vi "CleanUp.vi"(8 "error in (no error)":errorcluster, 11 "Prueba01 in":refnum<class "Prueba01.lvclass">) -> (0 "error out":errorcluster, 3 "Prueba01 out":refnum<class "Prueba01.lvclass">)   [LabVIEW 2019, in "Prueba01.lvclass"]
uses:
  Prueba01.lvclass
  C:/Users/ivan_/Documents/procal/Pruebas/Prueba/Prueba.lvclass
  Prueba/Prueba.lvclass/Prueba.ctl
  Prueba01.lvclass/Prueba01.ctl
  Base de Datos/SQLiteConnector/SQLiteConnection.lvclass
  Base de Datos/Base de Datos.lvclass
  Prueba/Prueba.lvclass
panel:
  # "estos daros\nse escribirán en la base de datos"
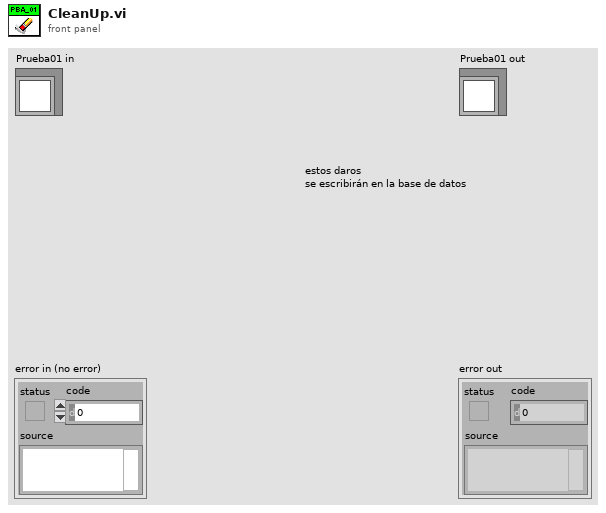
[diagram p1: front panel]
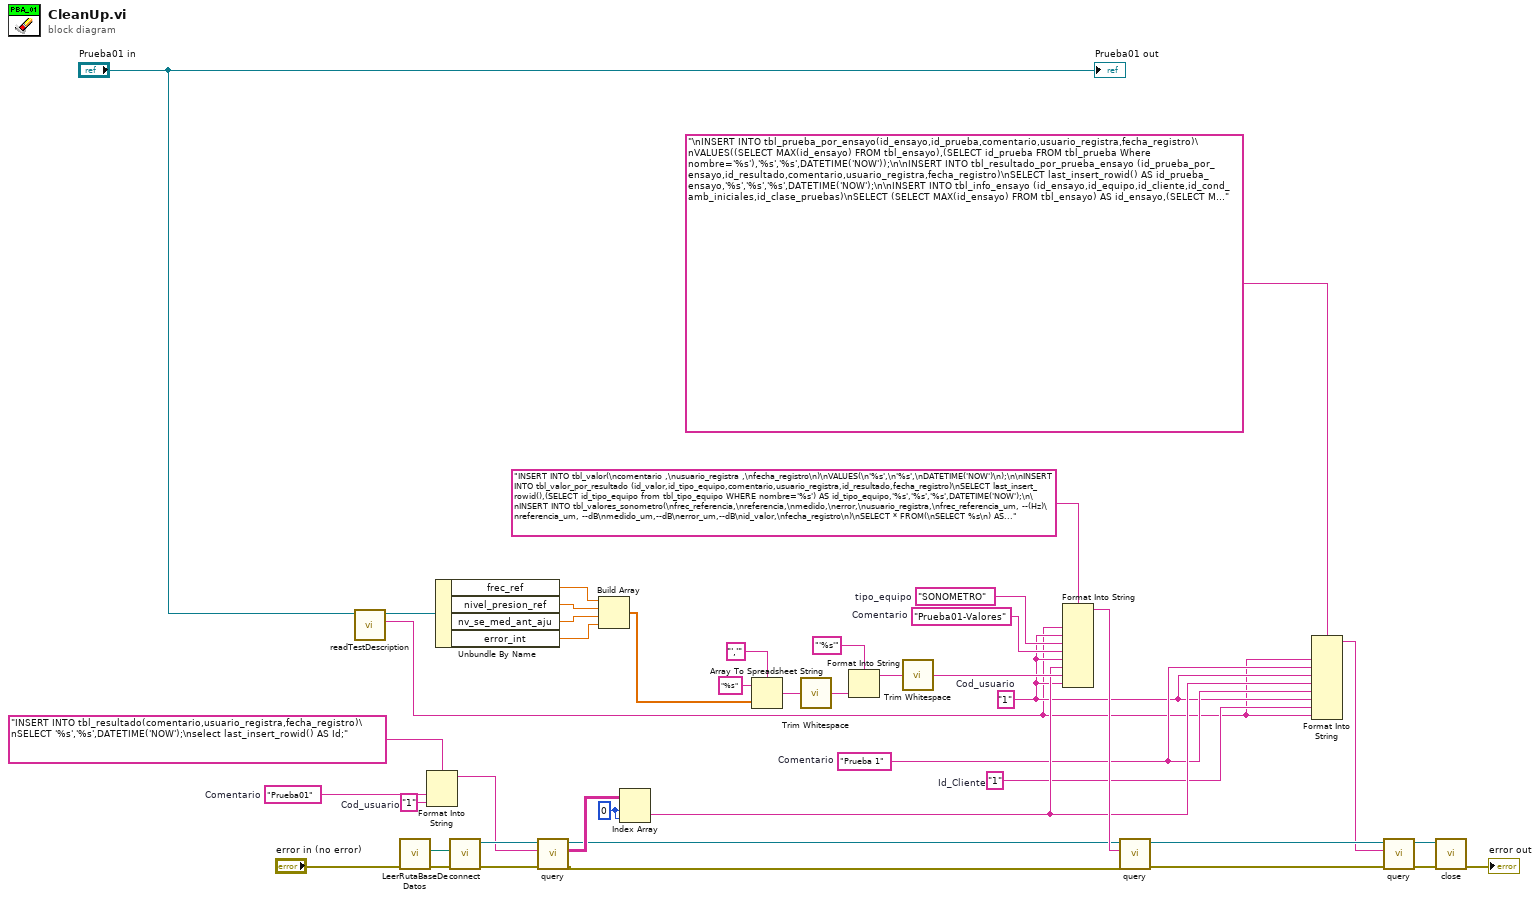
[diagram p0: block diagram]
diagram:
  w18 = "1"  # Id_Cliente
  w19 = "Prueba 1"  # Comentario
  w28 = "SONOMETRO"  # tipo_equipo
  w27 = "Prueba01-Valores"  # Comentario
  w34 = 0 ("index (row)")
  w36 = "1"  # Cod_usuario
  w37 = "Prueba01"  # Comentario
  w15 = "1"  # Cod_usuario
  n1 = call "readTestDescription.vi"("Prueba in"="Prueba01 in") -> ("Test Description"=w2:string, "Prueba out"=w1:refnum<class "Prueba01.lvclass">)  [unwired: 8 in, 1 out]
  n2 = call "LeerRutaBaseDeDatos.vi"("error in (no error)"="error in (no error)") -> ("error out"=w42:errorcluster, "Database Path"=w41:path)  [unwired: 9 in]
  n3 = Format Into String(format string="INSERT INTO tbl_resultado(comentario,usuario_registra,fecha_registro)\nSELECT '%s','%s',DATETIME('NOW');\nselect last_insert_rowid() AS Id;" ("SQL Statement"), w37, w36) -> (resulting string=w35:string)  [unwired: 2 in, 1 out]
  n4 = Unbundle By Name(w1) -> ("frec_ref"=w6:dbl, "nivel_presion_ref"=w7:dbl, "nv_se_med_ant_aju"=w8:dbl, "error_int"=w9:dbl)
  n5 = call "connect.vi"("error in (no error)"=w42, "Database Path"=w41) -> ("error out"=w33:errorcluster, "object out"=w39:refnum<class "SQLiteConnection.lvclass">)  [unwired: 8 in]
  n6 = call "query.vi"("error in (no error)"=w33, "SQL Statement"=w35, "object in"=w39) -> ("error out"=w30:errorcluster, "result"=w32:string[][], "object out"=w31:refnum<class "SQLiteConnection.lvclass">)  [unwired: 5 in, 1 out]
  n7 = Build Array(w6, w7, w8, w9) -> (w5:dbl[])
  n8 = Index Array(array=w32, index (row)=w34, index (col)=w34) -> (element=w20:string)
  n9 = Array To Spreadsheet String(delimiter (Tab)="','", array=w5, 3:"%s" ("format string")) -> (spreadsheet string=w11:string)
  n10 = call <vilib>:"Trim Whitespace.vi"("string"=w11) -> ("trimmed string"=w10:string)  [unwired: 1 in]
  n11 = Format Into String(format string="'%s'", w10) -> (resulting string=w4:string)  [unwired: 2 in, 1 out]
  n12 = call <vilib>:"Trim Whitespace.vi"("string"=w4) -> ("trimmed string"=w29:string)  [unwired: 1 in]
  n13 = Format Into String(format string="INSERT INTO tbl_valor(\ncomentario ,\nusuario_registra ,\nfecha_registro\n)\nVALUES(\n'%s',\n'%s',\nDATETIME('NOW')\n);\n\nINSERT INTO tbl_valor_por_resultado (id_valor,id_tipo_equipo,comentario,usuario_registra,id_resultado,fecha_registro)\nSELECT last_insert_rowid(),(SELECT id_tipo_equipo from tbl_tipo_equipo WHERE nombre='%s') AS id_tipo_equipo,'%s','%s','%s',DATETIME('NOW');\n\nINSERT INTO tbl_valores_sonometro(\nfrec_referencia,\nreferencia,\nmedido,\nerror,\nusuario_registra,\nfrec_referencia_um, --(Hz)\nreferencia_um, --dB\nmedido_um,--dB\nerror_um,--dB\nid_valor,\nfecha_registro\n)\nSELECT * FROM(\nSELECT %s\n) AS T\nINNER JOIN\n(SELECT %s AS usuario,'Hz','dB','dB','dB',(SELECT MAX(id_valor) FROM tbl_valor) AS id_valor,DATETIME('NOW') fecha ) AS F;", w2, w15, w28, w27, w15, w20, w29, w15) -> (resulting string=w40:string)  [unwired: 2 in, 1 out]
  n14 = call "query.vi"("error in (no error)"=w30, "SQL Statement"=w40, "object in"=w31) -> ("error out"=w24:errorcluster, "object out"=w26:refnum<class "SQLiteConnection.lvclass">)  [unwired: 5 in, 2 out]
  n15 = Format Into String(format string="\nINSERT INTO tbl_prueba_por_ensayo(id_ensayo,id_prueba,comentario,usuario_registra,fecha_registro)\nVALUES((SELECT MAX(id_ensayo) FROM tbl_ensayo),(SELECT id_prueba FROM tbl_prueba Where nombre='%s'),'%s','%s',DATETIME('NOW'));\n\nINSERT INTO tbl_resultado_por_prueba_ensayo (id_prueba_por_ensayo,id_resultado,comentario,usuario_registra,fecha_registro)\nSELECT last_insert_rowid() AS id_prueba_ensayo,'%s','%s','%s',DATETIME('NOW');\n\nINSERT INTO tbl_info_ensayo (id_ensayo,id_equipo,id_cliente,id_cond_amb_iniciales,id_clase_pruebas)\nSELECT (SELECT MAX(id_ensayo) FROM tbl_ensayo) AS id_ensayo,(SELECT MAX(id_equipo) FROM tbl_equipo) AS id_equipo,'%s' AS id_cliente,(SELECT MAX(id_cond_amb_iniciales) FROM tbl_cond_amb_iniciales) AS id_cond_amb_iniciales,\n(SELECT id_clase_prueba FROM tbl_clase_prueba WHERE id_clase=(SELECT id_clase FROM tbl_equipo ORDER BY id_equipo DESC LIMIT 1)  AND id_prueba=(SELECT id_prueba FROM tbl_prueba Where nombre='%s')) AS id_clase_pruebas;\n", w2, w19, w15, w20, w19, w15, w18, w2) -> (resulting string=w21:string)  [unwired: 2 in, 1 out]
  n16 = call "query.vi"("error in (no error)"=w24, "SQL Statement"=w21, "object in"=w26) -> ("error out"=w23:errorcluster, "object out"=w25:refnum<class "SQLiteConnection.lvclass">)  [unwired: 5 in, 2 out]
  n17 = call-dynamic "close.vi"("error in (no error)"=w23, "object in"=w25) -> ("error out"=→"error out":errorcluster)  [unwired: 8 in, 1 out]
  "Prueba01 out" <- "Prueba01 in"
